vi "Indicator_Error_Color.vi"(11 "AI 0":T1) -> (3 "Label.Text Colors:BG Color":u32)   [LabVIEW 2018]
uses:
  Controls/Clusts/ErrorStatus.ctl
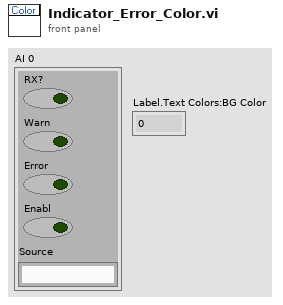
[diagram p1: front panel]
types:
  T1 = typedef "ErrorStatus.ctl" = cluster{"RX?":bool, "Warn":bool, "Error":bool, "Enabl":bool, "Source":string}
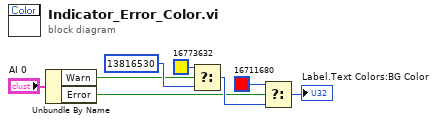
[diagram p0: block diagram]
diagram:
  n1 = Unbundle By Name("AI 0") -> ("Warn"=w1:bool, "Error"=w4:bool)
  n2 = Select(t=u32 16773632 ("Color Box"), s=w1, f=u32 13816530 ("Label.Text Colors:BG Color")) -> (s? t:f=w5:u32)
  n3 = Select(t=u32 16711680 ("Color Box 2"), s=w4, f=w5) -> (s? t:f=→"Label.Text Colors:BG Color":u32)
